vi "LoadValuesFromDash.vi"(8 "error in":errorcluster) -> (0 "error out":errorcluster)   [LabVIEW 2015]
uses:
  Drive/Implementation/Advanced Drive VIs/PID Type Def.ctl
  Motor Ref Names Type Def.ctl
  <vilib>/Rock Robotics/Network Tables/NT Read Numeric Array.vi
  Robot Global Data.vi
  <vilib>/Rock Robotics/Network Tables/NT Write Numeric Array.vi
  Drive/Implementation/RobotDriveGlobal.vi
panel:
  out "Numeric Array 2":dbl[](array[numeric])
  out "Numeric Array":dbl[](array[numeric])
  out "millisecond timer value":u32
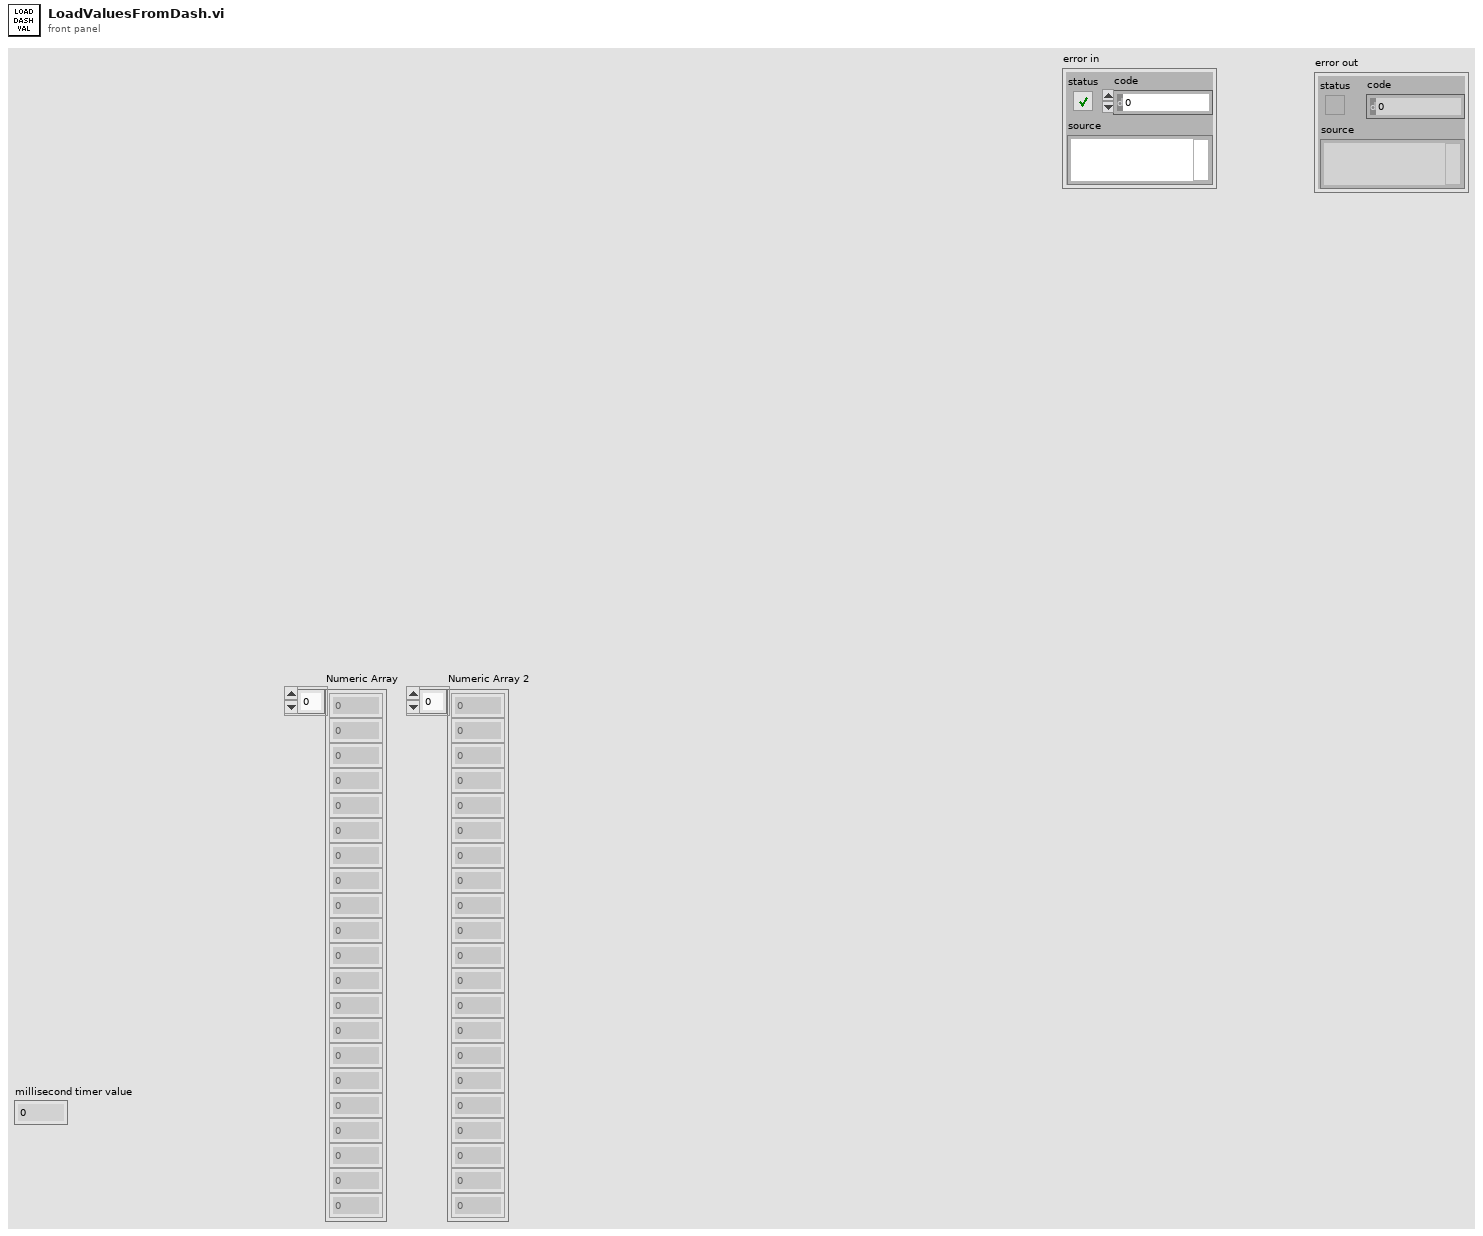
[diagram p1: front panel]
types:
  T1 = typedef "Robot Type Def.ctl" = enum32{"Disabled", "Ghost", "Casper", "Lofty", "Board"}
  T2 = typedef "PID Type Def.ctl" = cluster{"P":dbl, "I":dbl, "D":dbl, "F":dbl, "I Zone":dbl, "Ramp Rate":dbl}
  T3 = typedef "Motor Ref Names Type Def.ctl" = enum16{"Angular Motor", "Shooter Motor Bottom", "Shooter Motor Top", "Arm Shooter Motor"}
  T4 = typedef "Motor Ref Array Type Def.ctl" = T5[]
  T5 = typedef "Detailed Motor Type Def.ctl" = cluster{"MotorRef":T6, "Encoder Ticks Per Rev":dbl, "Set Position":dbl}
  T6 = typedef "WPI_MotorControlDeviceRef.ctl" = cluster{"DeviceStatus":errorcluster, "Type":T7, "PWM":cluster{"PWM Channel":T8, "DeadBand":T9}, "CAN":cluster{"Device Number":u8, "Control Mode":T10, "Semaphore":T11, "Max Vout":dbl, "TalonSRX Control Mode":T12}, "Invert":bool}
  T7 = typedef "WPI_MotorControlType.ctl" = enum16{"PWM", "CAN", "CANTalonSRX"}
  T8 = typedef "FPGA_DIOPWMChannel.ctl" = enum8{"PWM 0", "PWM 1", "PWM 2", "PWM 3", "PWM 4", "PWM 5", "PWM 6", "PWM 7", "PWM 8", "PWM 9", "PWM MXP 0", "PWM MXP 1", "PWM MXP 2", "PWM MXP 3", "PWM MXP 4", "PWM MXP 5", "PWM MXP 6", "PWM MXP 7", "PWM MXP 8", "PWM MXP 9", "Invalid"}
  T9 = typedef "WPI_PWMDeadband.ctl" = cluster{"Name":string, "maxPositivePwm":i32, "minPositivePwm":i32, "centerPwm":i32, "maxNegativePwm":i32, "minNegativePwm":i32, "angularRange":u16}
  T10 = typedef "WPI_CANJaguar_ControlMode.ctl" = enum8{"Percent VBus", "Current", "Speed", "Position", "Voltage"}
  T11 = typedef "Semaphore RefNum" = refnum<k1>
  T12 = typedef "WPI_CANTalonSRX_APIControlMode.ctl" = enum8{"Percent VBus", "Speed", "Position", "Slave", "Unchanged / Invalid", "Voltage Compensation", "Current", "Motion Profile"}
  T13 = typedef "RobotDrive Type Def.ctl" = cluster{"RobotDriveDevRef":cluster{"DevStatus":errorcluster, "Motors[]":T6[], "Square Inputs":bool, "Max Output":dbl}, "Control Mode":T12, "Motor Settings":T14, "Default Control Mode":T12}
  T14 = typedef "Drive Motor Settings.ctl" = cluster{"Wheel Radius":dbl, "Encoder Ticks Per Rev":dbl, "Gear Ratio":dbl, "ClimbRev":dbl}
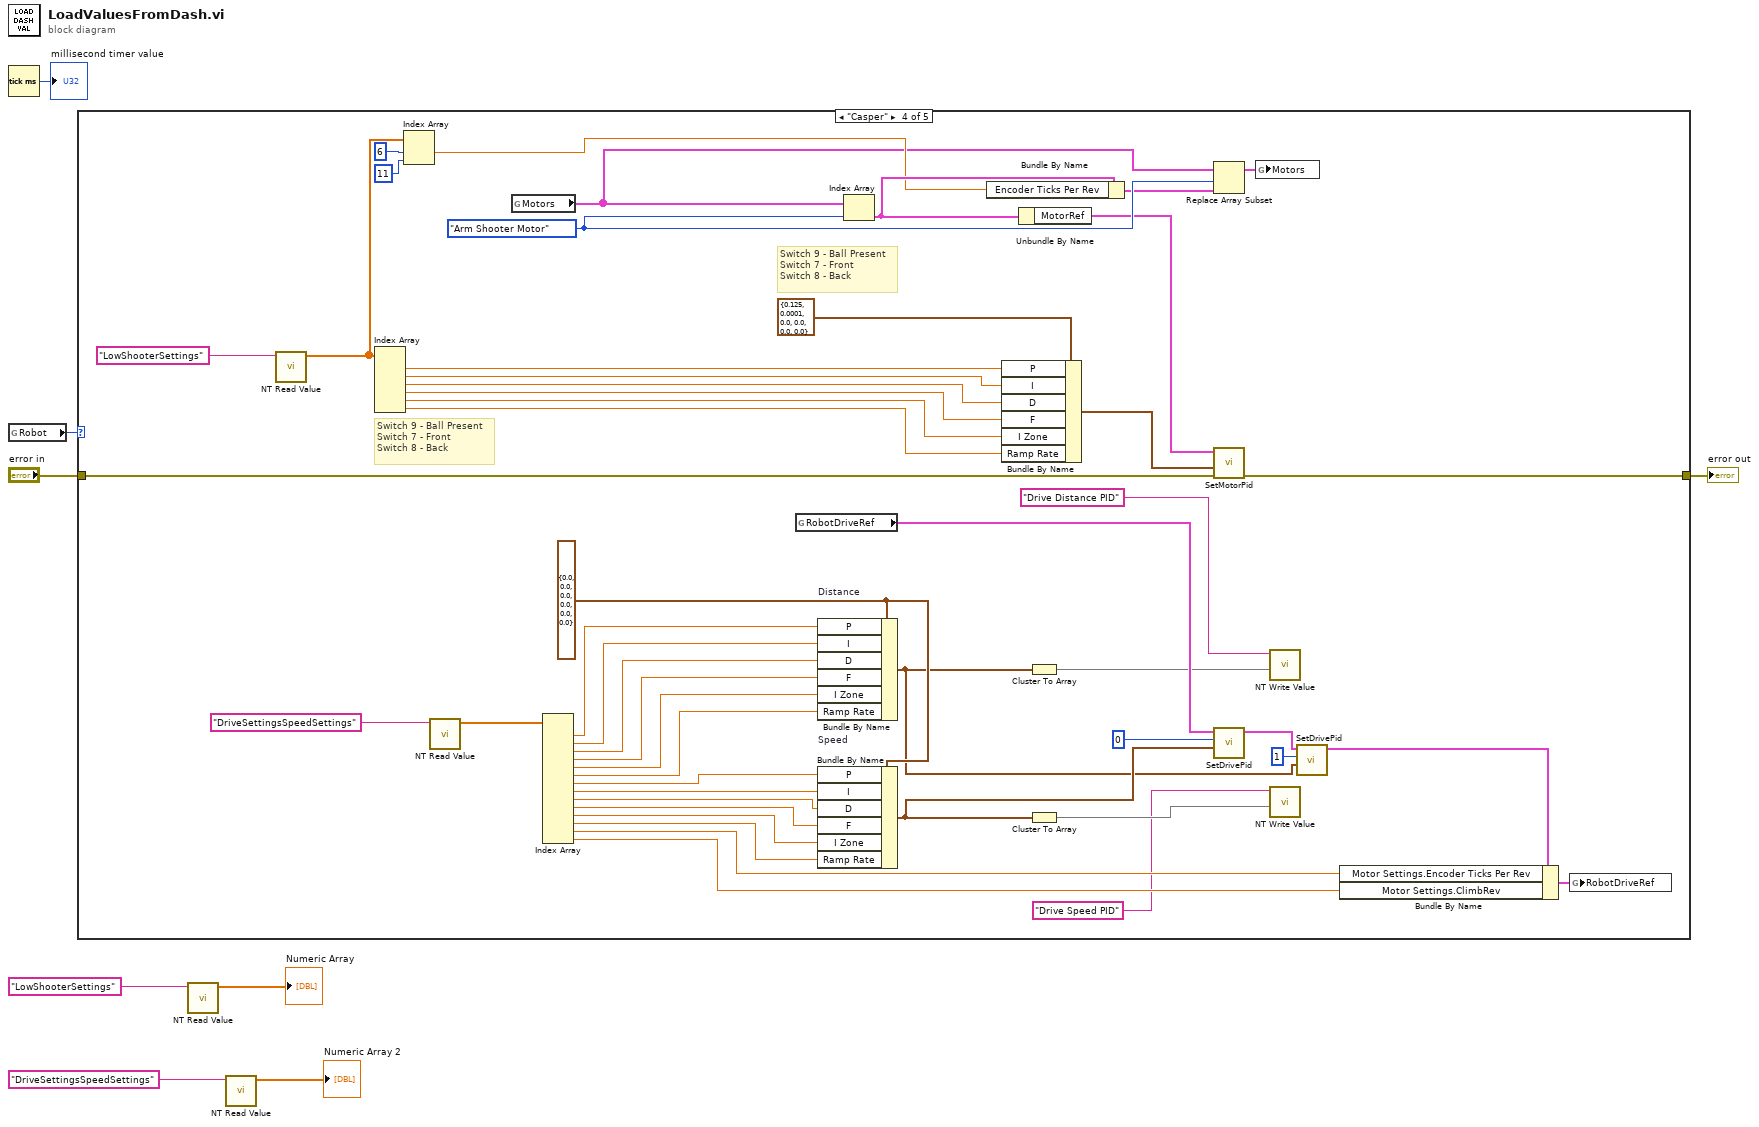
[diagram p0: block diagram]
diagram:
  n1 = Tick Count (ms)() -> (millisecond timer value=→"millisecond timer value":u32)
  n2 = global read "Robot Global Data.vi" "Robot"() -> (w8:T1)
  n3 = case shown="\"Casper\"" w8 {
    tunnel: [w9 w10 w11 w52 w62] -> w7
    tunnel: "error in" -> [w9 w10 w11 w41 w62]
    frame "Disabled", Default {
    }
    frame "Board" {
    }
    frame "Ghost" {
    }
    frame "Casper" {
      w32 = T2 {"P"=0.0, "I"=0.0, "D"=0.0, "F"=0.0, "I Zone"=0.0, "Ramp Rate"=0.0} ("PID")
      w45 = Motor_Ref_Names_Type_Def."Arm Shooter Motor" ("Motor Ref Names")
      # "Switch 9 - Ball Present\nSwitch 7 - Front\nSwitch 8 - Back"
      # "Switch 9 - Ball Present\nSwitch 7 - Front\nSwitch 8 - Back"
      n4 = call-poly <vilib>:"NT Read Value.vi"("Name"="LowShooterSettings") -> ("Numeric Array"=w49:dbl[])  [unwired: 9 in, 1 out]
      n5 = Index Array(array=w49) -> (element #1=w59:dbl, element #2=w58:dbl, element #3=w57:dbl, element #4=w56:dbl, element #5=w55:dbl, element #6=w54:dbl)  [unwired: 6 in]
      n6 = Index Array(array=w49, index #1=6 ("index"), index #2=11 ("index")) -> (element #1=w47:dbl)  [unwired: 1 out]
      n7 = call-poly <vilib>:"NT Read Value.vi"("Name"="DriveSettingsSpeedSettings") -> ("Numeric Array"=w39:dbl[])  [unwired: 9 in, 1 out]
      n8 = global read "Robot Global Data.vi" "Motors"() -> (w46:T4)
      n9 = Index Array(array=w39) -> (element #1=w38:dbl, element #2=w37:dbl, element #3=w36:dbl, element #4=w35:dbl, element #5=w34:dbl, element #6=w33:dbl, element #7=w31:dbl, element #8=w30:dbl, element #9=w29:dbl, element #10=w28:dbl, element #11=w27:dbl, element #12=w26:dbl, element #13=w18:dbl, element #14=w19:dbl)  [unwired: 14 in]
      n10 = global read "RobotDriveGlobal.vi" "RobotDriveRef"() -> (w25:T13)
      n11 = Bundle By Name "Distance"(cluster=w32, "P"=w38, "I"=w37, "D"=w36, "F"=w35, "I Zone"=w34, "Ramp Rate"=w33) -> (w16:T2)
      n12 = Bundle By Name "Speed"(cluster=w32, "P"=w31, "I"=w30, "D"=w29, "F"=w28, "I Zone"=w27, "Ramp Rate"=w26) -> (w17:T2)
      n13 = Index Array(array=w46, index=w45) -> (element=w48:T5)
      n14 = Bundle By Name(cluster=w48, "Encoder Ticks Per Rev"=w47) -> (w44:T5)
      n15 = Bundle By Name(cluster=T2 {"P"=0.125, "I"=0.0001, "D"=0.0, "F"=0.0, "I Zone"=0.0, "Ramp Rate"=0.0} ("PID"), "P"=w59, "I"=w58, "D"=w57, "F"=w56, "I Zone"=w55, "Ramp Rate"=w54) -> (w53:T2)
      n16 = Unbundle By Name(w48) -> ("MotorRef"=w42:T6)
      n17 = Cluster To Array(cluster=w16) -> (array=w13:dbl[])
      n18 = Cluster To Array(cluster=w17) -> (array=w15:dbl[])
      n19 = Replace Array Subset(array=w46, new element=w44, index=w45) -> (w43:T4)
      n20 = call "SetMotorPid.vi"("error in (no error)"=w41, "PID"=w53, "Motor Ref In"=w42) -> ("error out"=w52:errorcluster)  [unwired: 7 in, 1 out]
      n21 = call "SetDrivePid.vi"("PID"=w17, "Profile Slot"=u8 0, "RobotDriveRef In"=w25) -> ("RobotDriveRef Out"=w23:T13)  [unwired: 7 in, 1 out]
      n22 = global write "Robot Global Data.vi" "Motors"(w43) -> ()
      n23 = call-poly <vilib>:"NT Write Value.vi"("Numeric Array"=w13, "Name"="Drive Distance PID") -> ()  [unwired: 9 in, 1 out]
      n24 = call-poly <vilib>:"NT Write Value.vi"("Numeric Array"=w15, "Name"="Drive Speed PID") -> ()  [unwired: 9 in, 1 out]
      n25 = call "SetDrivePid.vi"("PID"=w16, "Profile Slot"=u8 1, "RobotDriveRef In"=w23) -> ("RobotDriveRef Out"=w21:T13)  [unwired: 7 in, 1 out]
      n26 = Bundle By Name(cluster=w21, "Motor Settings.Encoder Ticks Per Rev"=w18, "Motor Settings.ClimbRev"=w19) -> (w20:T13)
      n27 = global write "RobotDriveGlobal.vi" "RobotDriveRef"(w20) -> ()
    }
    frame "Lofty" {
    }
  }
  "error out" <- w7
  n28 = call-poly <vilib>:"NT Read Value.vi"("Name"="LowShooterSettings") -> ("Numeric Array"=→"Numeric Array":dbl[])  [unwired: 9 in, 1 out]
  n29 = call-poly <vilib>:"NT Read Value.vi"("Name"="DriveSettingsSpeedSettings") -> ("Numeric Array"=→"Numeric Array 2":dbl[])  [unwired: 9 in, 1 out]
